vi "Main.vi"() -> ()   [LabVIEW 2014]
uses:
  <vilib>/Utility/sysdir.llb/System Directory Type.ctl
panel:
  out "Application:Kind":T1(ring)
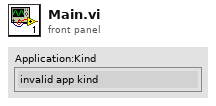
[diagram p1: front panel]
types:
  T1 = enum32{"invalid app kind", "Development System", "Run Time System", "Student Edition", "Embedded LabVIEW", "Evaluation", "Custom"}
  T2 = typedef "System Directory Type.ctl" = i32
  T3 = enum16{"open", "replace", "create", "open or create", "replace or create", "replace or create with confirmation"}
  T4 = cluster{"Team Number":string, "Autonomous?":string, "Autonomous Comments":string, "Did they start in \nthe goalie zone??":string, "Top Goal":dbl, "Bottom Goal":dbl, "Did they move?":string, "Was the goal lit?":string}
  T5 = cluster{"Team Number":string, "Autonomous?":string, "Autonomous Comments":string, "Did they start in \nthe goalie zone??":string, dbl, dbl, "Did they move?":string, "Was the goal lit?":string}
  T6 = cluster{"Top Goal":dbl, "Bottom Goal":dbl, "Missed Shots":dbl, "Total":dbl, "Helps":dbl, "Over Truss With Catch":dbl, "Over the Truss Pass":dbl, "Under the Truss Pass":dbl, "Can they pick up the ball?":string, "Can they catch?":string, "Defense?":string, "Comments":string}
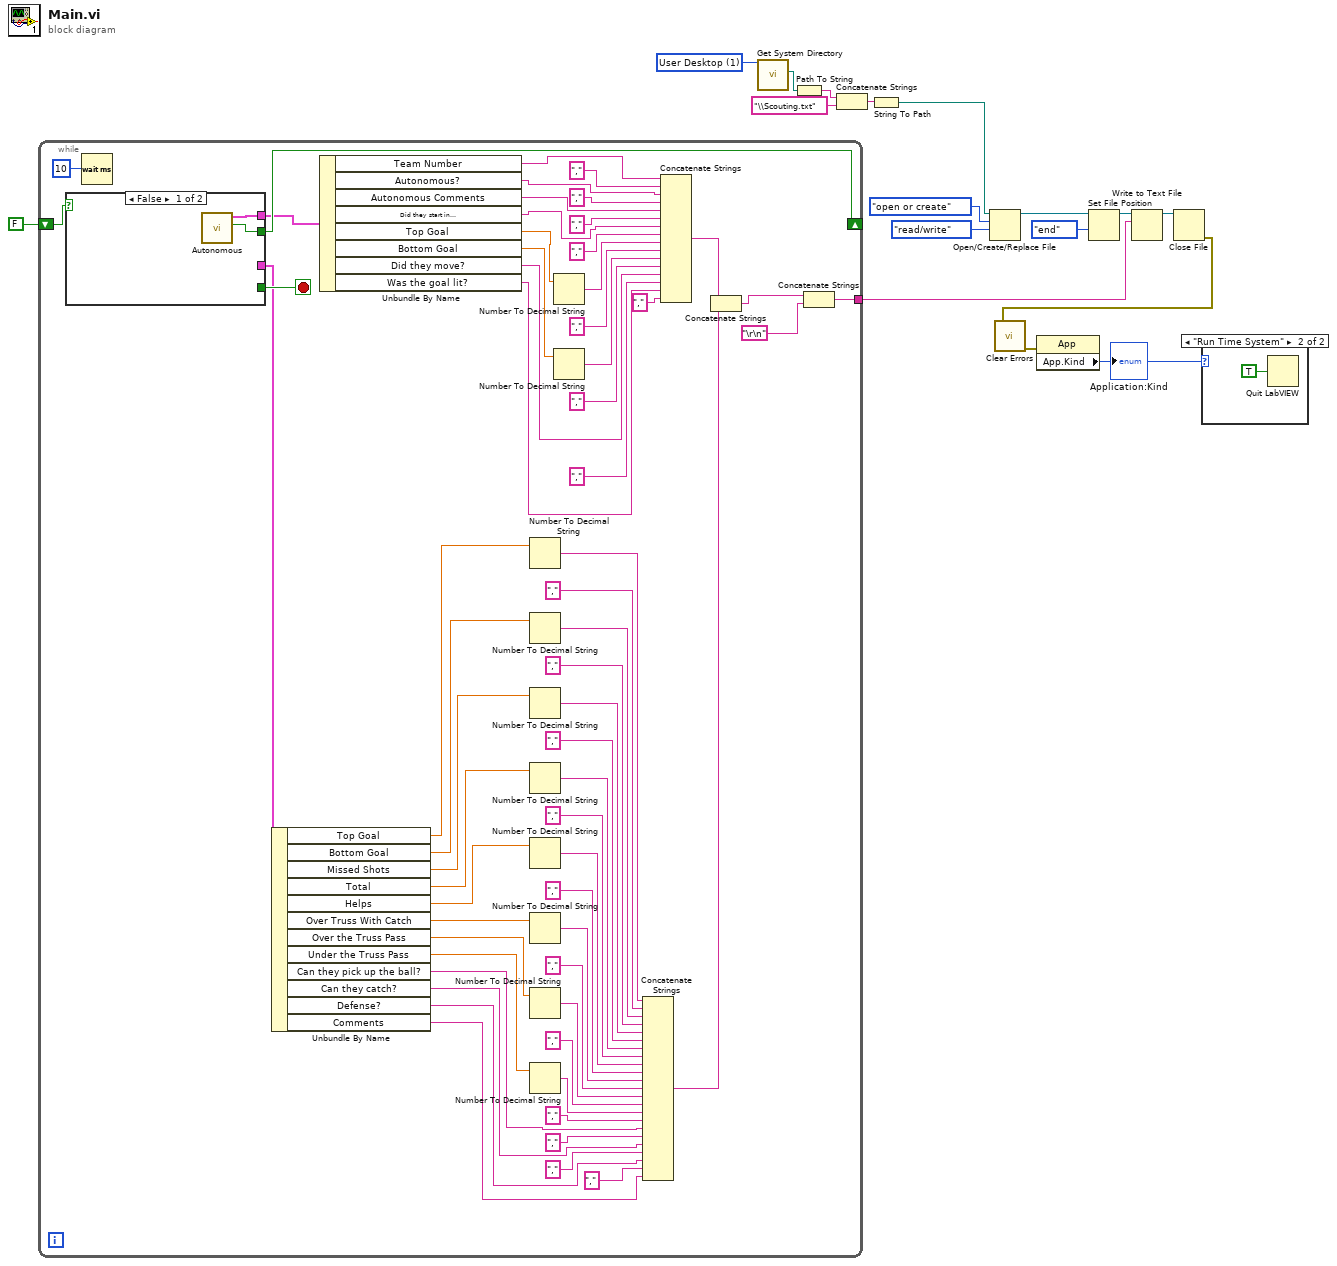
[diagram p0: block diagram]
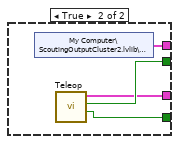
[diagram p3: hidden frame]
diagram:
  w2 = T2 1 items=["User Home"=0, "User Desktop"=1, "User Documents"=2, "User Application Data"=3, "User Preferences"=4, "User Temporary"=5, "Public Documents"=6, "Public Application Data"=7, "Public Preferences"=8, "Public Cache"=13, "System Core Libraries"=9, "System Installed Libraries"=10, "Application Files"=11, "Boot Volume Root"=12] ("system directory type")
  n1 = while {
    shift-right: [w75] -> _
    shift-left: FALSE ("Boolean") -> [w76]
    tunnel: [w43] -> w10
    stop <- w74 stop-if-true
    n2 = case shown="False" w76 {
      tunnel: [w79 w82] -> w75
      tunnel: [w78 w80] -> w42
      tunnel: [_ w83] -> w74
      tunnel: [_ w81] -> w33
      frame False {
        n3 = call "Autonomous.vi"() -> ("Switch To Teleop"=w79:bool, "output cluster"=w78:T4)  [unwired: 10 in]
      }
      frame True {
        n4 = shared-variable "My Computer\\ScoutingOutputCluster2.lvlib\\output cluster"() -> (w80:T5)  [unwired: 1 in, 1 out]
        n5 = call "Teleop.vi"() -> ("Stop program and write to file"=w83:bool, "SWITCH TO AUTONOMOUS 2"=w82:bool, "output cluster"=w81:T6)  [unwired: 9 in]
      }
    }
    n6 = Wait (ms)(milliseconds to wait=u32 10) -> ()  [unwired: 1 out]
    n7 = Unbundle By Name(w33) -> ("Top Goal"=w32:dbl, "Bottom Goal"=w31:dbl, "Missed Shots"=w30:dbl, "Total"=w29:dbl, "Helps"=w28:dbl, "Over Truss With Catch"=w27:dbl, "Over the Truss Pass"=w26:dbl, "Under the Truss Pass"=w25:dbl, "Can they pick up the ball?"=w24:string, "Can they catch?"=w23:string, "Defense?"=w22:string, "Comments"=w20:string)
    n8 = Unbundle By Name(w42) -> ("Team Number"=w41:string, "Autonomous?"=w40:string, "Autonomous Comments"=w39:string, "Did they start in \nthe goalie zone??"=w38:string, "Top Goal"=w37:dbl, "Bottom Goal"=w36:dbl, "Did they move?"=w35:string, "Was the goal lit?"=w34:string)
    n9 = Number To Decimal String(number=w32) -> (decimal integer string=w63:string)  [unwired: 1 in]
    n10 = Number To Decimal String(number=w31) -> (decimal integer string=w61:string)  [unwired: 1 in]
    n11 = Number To Decimal String(number=w30) -> (decimal integer string=w59:string)  [unwired: 1 in]
    n12 = Number To Decimal String(number=w29) -> (decimal integer string=w57:string)  [unwired: 1 in]
    n13 = Number To Decimal String(number=w28) -> (decimal integer string=w55:string)  [unwired: 1 in]
    n14 = Number To Decimal String(number=w27) -> (decimal integer string=w53:string)  [unwired: 1 in]
    n15 = Number To Decimal String(number=w26) -> (decimal integer string=w51:string)  [unwired: 1 in]
    n16 = Number To Decimal String(number=w25) -> (decimal integer string=w49:string)  [unwired: 1 in]
    n17 = Number To Decimal String(number=w37) -> (decimal integer string=w69:string)  [unwired: 1 in]
    n18 = Number To Decimal String(number=w36) -> (decimal integer string=w67:string)  [unwired: 1 in]
    n19 = Concatenate Strings(w63, "," ("string"), w61, "," ("string"), w59, "," ("string"), w57, "," ("string"), w55, "," ("string"), w53, "," ("string"), w51, "," ("string"), w49, "," ("string"), w24, "," ("string"), w23, "," ("string"), w22, "," ("string"), w20) -> (w44:string)
    n20 = Concatenate Strings(w41, "," ("string"), w40, "," ("string"), w39, "," ("string"), w38, "," ("string"), w69, "," ("string"), w67, "," ("string"), w35, "," ("string"), w34, "," ("string")) -> (w45:string)
    n21 = Concatenate Strings(w45, w44) -> (w19:string)
    n22 = Concatenate Strings(w19, "\r\n") -> (w43:string)
  }
  n23 = call <vilib>:"Get System Directory.vi"("system directory type"=w2) -> ("system directory"=w6:path)  [unwired: 10 in]
  n24 = Path To String(path=w6) -> (string=w5:string)
  n25 = Concatenate Strings(w5, "\\Scouting.txt" ("string")) -> (w4:string)
  n26 = String To Path(string=w4) -> (path=w1:path)
  n27 = Open/Create/Replace File(file path (use dialog)=w1, operation (0:open)=T3."open or create", access (0:read/write)=enum16{"read/write", "read-only", "write-only"}."read/write") -> (refnum out=w15:refnum<file>)  [unwired: 3 in, 2 out]
  n28 = Set File Position(refnum=w15, from (0:start)=enum16{"start", "end", "current"}."end") -> (refnum out=w16:refnum<file>)  [unwired: 2 in, 1 out]
  n29 = Write to Text File(file (use dialog)=w16, text=w10) -> (refnum out=w13:refnum<file>)  [unwired: 2 in, 2 out]
  n30 = Close File(refnum=w13) -> (error out=w7:errorcluster)  [unwired: 1 in, 1 out]
  n31 = call <vilib>:"Clear Errors.vi"("error in (no error)"=w7) -> ("error out"=w8:errorcluster)  [unwired: 5 in, 1 out]
  n32 = property class="App"(error in=w8) -> ("App.Kind"=w9:T1)  [unwired: 1 in, 2 out]
  "Application:Kind" <- w9
  n33 = case shown="\"Run Time System\"" w9 {
    frame Default {
    }
    frame "Run Time System" {
      n34 = Quit LabVIEW(quit? (T)=TRUE) -> ()
    }
  }
